vi "Maxi Gauge-Data-Display control.vi"(0 "VISA-Ressource in":refnum<visa-resource-name>, 1 "Node address":i8=-1 min=-1 max=31 step=1, 2 "W/R":bool, 5 "Baragraph Set":i8(ring)=3 items=["off", "Sensor-Range", "1 Decade", ""], 7 "Digits Set":i8(ring)=4 items=["", "", "2", "3", ""], 9 "Unit Set":i8(ring)=4 items=["mbar", "Torr", "Pascal", "", ""], 11 "Fehler (Eingang)":errorcluster) -> (4 "VISA-Ressource out":refnum<visa-resource-name>, 6 "Baragraph Get":i8(ring)=1 items=["off", "Sensor-Range", "1 Decade", ""], 8 "Digits Get":i8(ring)=1 items=["", "", "2", "3", ""], 10 "Unit Get":i8(ring)=1 items=["mbar", "Torr", "Pascal", "", ""], 15 "Fehler (Ausgang)":errorcluster)   [LabVIEW 2012, in "Maxi Gauge.lvlib"]
uses:
  Maxi Gauge.lvlib
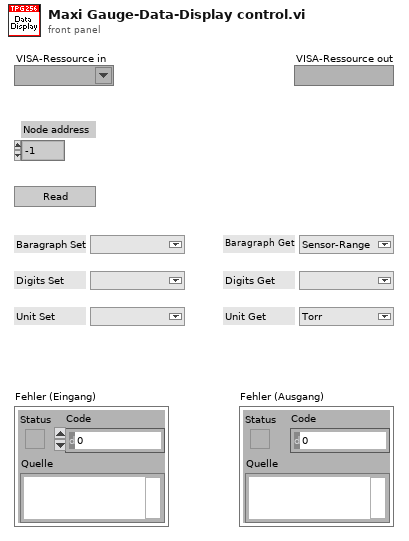
[diagram p1: front panel]
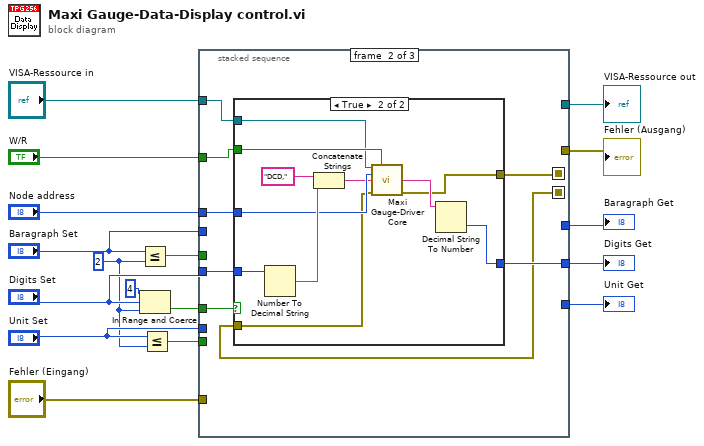
[diagram p0: block diagram]
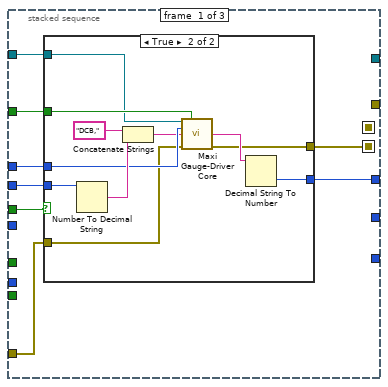
[diagram p2: hidden frame]
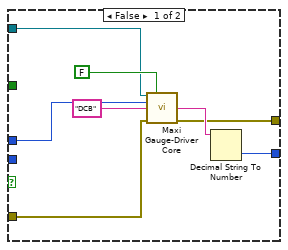
[diagram p3: hidden frame]
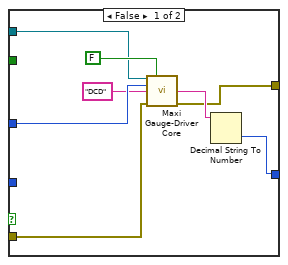
[diagram p4: hidden frame]
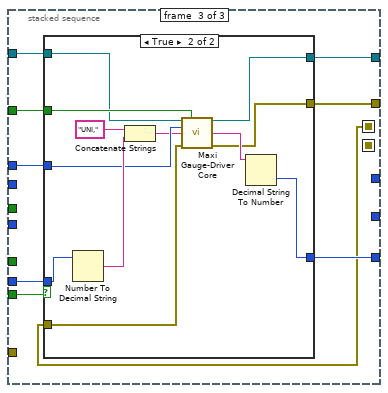
[diagram p5: hidden frame]
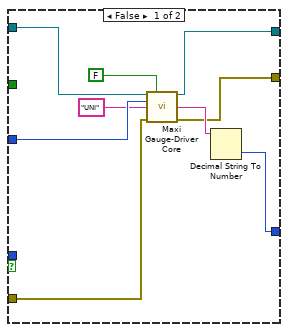
[diagram p6: hidden frame]
diagram:
  w1 = i8 2 ("y")
  n1 = Less Or Equal?(x="Baragraph Set", y=w1) -> (x <= y?=w7:bool)
  n2 = In Range and Coerce(upper limit=i8 4 ("hi"), x="Digits Set", lower limit=w1) -> (In Range?=w8:bool)  [unwired: 1 out]
  n3 = Less Or Equal?(x="Unit Set", y=w1) -> (x <= y?=w6:bool)
  n4 = stacked-sequence {
    seq-local: [w18 _ _] -> [_ w46 _]
    seq-local: [_ w45 _] -> [_ _ w73]
    tunnel: "W/R" -> [w25 w52 w80]
    tunnel: "Node address" -> [w24 w51 w79]
    tunnel: w7 -> [w23 _ _]
    tunnel: "Baragraph Set" -> [w22 _ _]
    tunnel: [w21 _ _] -> w13
    tunnel: "Digits Set" -> [_ w50 _]
    tunnel: w8 -> [_ w49 _]
    tunnel: [_ w48 _] -> w12
    tunnel: [_ _ w78] -> w11
    tunnel: w6 -> [_ _ w77]
    tunnel: "Unit Set" -> [_ _ w76]
    tunnel: "VISA-Ressource in" -> [w20 w47 w75]
    tunnel: [_ _ w74] -> w4
    tunnel: "Fehler (Eingang)" -> [w19 _ _]
    tunnel: [_ _ w72] -> w2
    frame #0 {
      n5 = case shown="True" w23 {
        tunnel: w25 -> [_ w43]
        tunnel: [w32 w40] -> w18
        tunnel: w24 -> [w31 w37]
        tunnel: w22 -> [_ w39]
        tunnel: [w30 w38] -> w21
        tunnel: w20 -> [w27 w35]
        tunnel: w19 -> [w28 w34]
        frame False {
          n6 = call "Maxi Gauge-Driver Core.vi"("VISA-Ressource in"=w27, "Write/Read"=FALSE, "Node address"=w31, "Command"="DCB", "Fehler (Eingang)"=w28) -> ("String Out"=w33:string, "Fehler (Ausgang)"=w32:errorcluster)  [unwired: 8 in, 1 out]
          n7 = Decimal String To Number(string=w33) -> (number=w30:i32)  [unwired: 2 in, 1 out]
        }
        frame True {
          n8 = Number To Decimal String(number=w39) -> (decimal integer string=w42:string)  [unwired: 1 in]
          n9 = Concatenate Strings("DCB,", w42) -> (w36:string)
          n10 = call "Maxi Gauge-Driver Core.vi"("VISA-Ressource in"=w35, "Write/Read"=w43, "Node address"=w37, "Command"=w36, "Fehler (Eingang)"=w34) -> ("String Out"=w44:string, "Fehler (Ausgang)"=w40:errorcluster)  [unwired: 8 in, 1 out]
          n11 = Decimal String To Number(string=w44) -> (number=w38:i32)  [unwired: 2 in, 1 out]
        }
      }
    }
    frame #1 {
      n12 = case shown="True" w49 {
        tunnel: w52 -> [_ w70]
        tunnel: [w59 w67] -> w45
        tunnel: w51 -> [w58 w64]
        tunnel: w50 -> [_ w66]
        tunnel: [w57 w65] -> w48
        tunnel: w47 -> [w55 w61]
        tunnel: w46 -> [w53 w63]
        frame False {
          n13 = call "Maxi Gauge-Driver Core.vi"("VISA-Ressource in"=w55, "Write/Read"=FALSE, "Node address"=w58, "Command"="DCD", "Fehler (Eingang)"=w53) -> ("String Out"=w60:string, "Fehler (Ausgang)"=w59:errorcluster)  [unwired: 8 in, 1 out]
          n14 = Decimal String To Number(string=w60) -> (number=w57:i32)  [unwired: 2 in, 1 out]
        }
        frame True {
          n15 = Number To Decimal String(number=w66) -> (decimal integer string=w69:string)  [unwired: 1 in]
          n16 = Concatenate Strings("DCD,", w69) -> (w62:string)
          n17 = call "Maxi Gauge-Driver Core.vi"("VISA-Ressource in"=w61, "Write/Read"=w70, "Node address"=w64, "Command"=w62, "Fehler (Eingang)"=w63) -> ("String Out"=w71:string, "Fehler (Ausgang)"=w67:errorcluster)  [unwired: 8 in, 1 out]
          n18 = Decimal String To Number(string=w71) -> (number=w65:i32)  [unwired: 2 in, 1 out]
        }
      }
    }
    frame #2 {
      n19 = case shown="True" w77 {
        tunnel: w80 -> [_ w100]
        tunnel: [w88 w97] -> w72
        tunnel: w79 -> [w87 w95]
        tunnel: [w86 w96] -> w78
        tunnel: w76 -> [_ w94]
        tunnel: w75 -> [w83 w92]
        tunnel: [w82 w91] -> w74
        tunnel: w73 -> [w81 w90]
        frame False {
          n20 = call "Maxi Gauge-Driver Core.vi"("VISA-Ressource in"=w83, "Write/Read"=FALSE, "Node address"=w87, "Command"="UNI", "Fehler (Eingang)"=w81) -> ("VISA-Ressource out"=w82:refnum<visa-resource-name>, "String Out"=w89:string, "Fehler (Ausgang)"=w88:errorcluster)  [unwired: 8 in]
          n21 = Decimal String To Number(string=w89) -> (number=w86:i32)  [unwired: 2 in, 1 out]
        }
        frame True {
          n22 = Number To Decimal String(number=w94) -> (decimal integer string=w99:string)  [unwired: 1 in]
          n23 = Concatenate Strings("UNI,", w99) -> (w93:string)
          n24 = call "Maxi Gauge-Driver Core.vi"("VISA-Ressource in"=w92, "Write/Read"=w100, "Node address"=w95, "Command"=w93, "Fehler (Eingang)"=w90) -> ("VISA-Ressource out"=w91:refnum<visa-resource-name>, "String Out"=w101:string, "Fehler (Ausgang)"=w97:errorcluster)  [unwired: 8 in]
          n25 = Decimal String To Number(string=w101) -> (number=w96:i32)  [unwired: 2 in, 1 out]
        }
      }
    }
  }
  "Baragraph Get" <- w13
  "Digits Get" <- w12
  "Unit Get" <- w11
  "VISA-Ressource out" <- w4
  "Fehler (Ausgang)" <- w2
